vi "CIMAQ_PM_UEP.vi"(8 "error in (no error)":errorcluster, 11 "Refnum in":T1) -> (0 "error out":errorcluster, 1 "Centroid":cluster{"X Centroid":sgl, "Y Centroid":sgl} {"Y Centroid" format="%.2f"; "X Centroid" format="%.2f"}, 2 "UEPs":cluster{i32, i32}[](array[cluster]), 3 "UEP":cluster{i32, i32})   [LabVIEW 2017]
uses:
  <vilib>/vision/Image Controls.llb/IMAQ Image.ctl
  <vilib>/vision/NI_Vision_Development_Module.lvlib
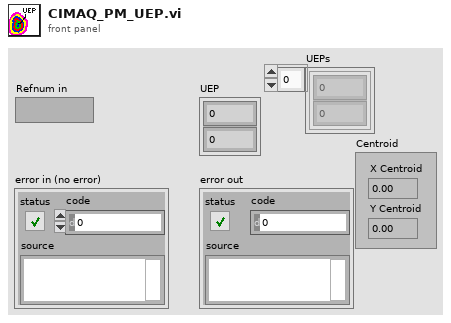
[diagram p1: front panel]
types:
  T1 = typedef "IMAQ Image.ctl" = refnum<image>
  T2 = typedef "Image Type" = u32
  T3 = cluster{"histogram":u32[], "Minimal Value":sgl, "Maximal Value":sgl, "Starting Value":sgl, "Interval Width":sgl, "Mean Value":sgl, "Standard  Variation":sgl, "Area (pixels)":i32}
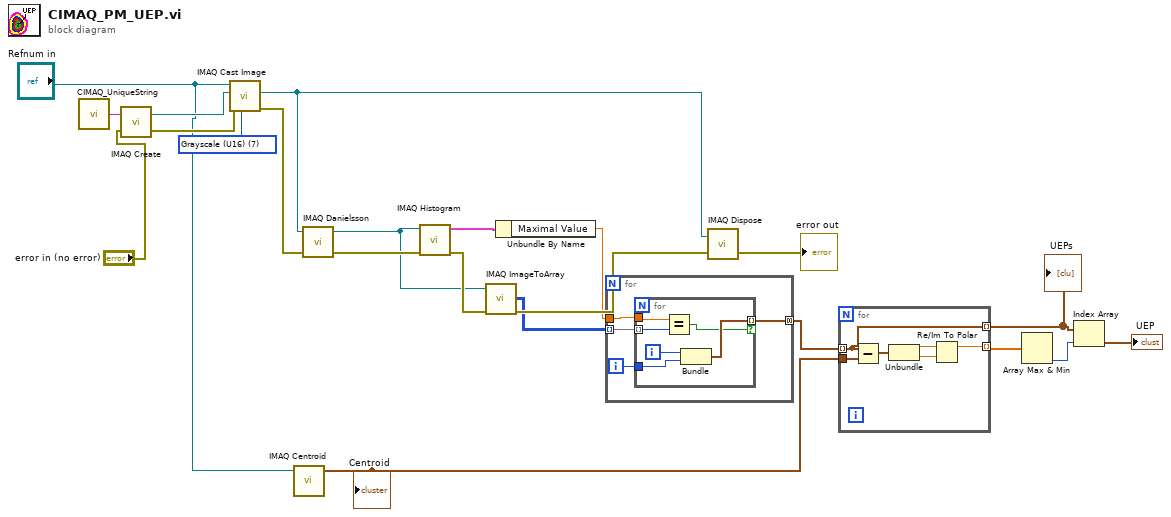
[diagram p0: block diagram]
diagram:
  w14 = T2 7 items=["Grayscale (U8)", "Grayscale (I16)", "Grayscale (SGL)", "Complex (CSG)", "RGB (U32)", "HSL (U32)", "RGB (U64)", "Grayscale (U16)"] ("Image Type")
  n1 = call <userlib>:"CIMAQ_UniqueString.vi"() -> ("String"=w18:string)  [unwired: 5 in]
  n2 = call "IMAQ Create"("Image Name"=w18, "error in (no error)"="error in (no error)") -> ("New Image"=w15:T1, "error out"=w11:errorcluster)  [unwired: 3 in]
  n3 = call "IMAQ Cast Image"("Image Type"=w14, "error in (no error)"=w11, "Image Dst"=w15, "Image Src"="Refnum in") -> ("error out"=w10:errorcluster, "Image Dst Out"=w13:T1)  [unwired: 6 in]
  n4 = call "IMAQ Centroid"("Image"="Refnum in") -> ("Centroid"=w5:cluster{"X Centroid":sgl, "Y Centroid":sgl})  [unwired: 3 in, 1 out]
  "Centroid" <- w5
  n5 = call "IMAQ Danielsson"("error in (no error)"=w10, "Image Src"=w13) -> ("error out"=w19:errorcluster, "Image Dst Out"=w17:T1)  [unwired: 2 in]
  n6 = call "IMAQ Histogram"("error in (no error)"=w19, "Image"=w17) -> ("error out"=w20:errorcluster, "Histogram Report"=w16:T3)  [unwired: 8 in]
  n7 = call "IMAQ ImageToArray"("error in (no error)"=w20, "Image"=w17) -> ("Image Pixels (U16)"=w7:u16[][], "error out"=w21:errorcluster)  [unwired: 2 in, 3 out]
  n8 = Unbundle By Name(w16) -> ("Maximal Value"=w8:sgl)
  n9 = for {
    tunnel: w8 -> [w26]
    tunnel: w7 -> [w25] mode=indexing
    tunnel: [w23] -> w6 mode=concatenating
    i -> [w24]
    n10 = for {
      tunnel: w26 -> [w32]
      tunnel: w25 -> [w31] mode=indexing
      tunnel: w24 -> [w29]
      tunnel: [w28] -> w23 mode=indexing if=w27
      i -> [w30]
      n11 = Equal?(x=w32, y=w31) -> (x = y?=w27:bool)
      n12 = Bundle(w30, w29) -> (w28:cluster{i32, i32})  [unwired: 1 in]
    }
  }
  n13 = call "IMAQ Dispose"("Image"=w13, "error in (no error)"=w21) -> ("error out"=→"error out":errorcluster)  [unwired: 4 in]
  n14 = for {
    tunnel: w6 -> [w33] mode=indexing
    tunnel: w5 -> [w38]
    tunnel: [w34] -> w4 mode=indexing
    tunnel: [w33] -> w2 mode=indexing
    n15 = Subtract(x=w33, y=w38) -> (x-y=w37:cluster{sgl, sgl})
    n16 = Unbundle(w37) -> (w35:sgl, w36:sgl)
    n17 = Re/Im To Polar(2:w36, 3:w35) -> (1:w34:sgl)  [unwired: 1 out]
  }
  "UEPs" <- w2
  n18 = Array Max & Min(array=w4) -> (min index (indices)=w3:i32)  [unwired: 3 out]
  n19 = Index Array(array=w2, index=w3) -> (element=→"UEP":cluster{i32, i32})
